vi "filterField.vi"(4 "Lado":enum16{"Esquerdo", "Direito"}(ring)=enum."Direito" caption="Enum", 5 "ignora esquerda?":bool=TRUE, 6 "Time":enum16{"Azul", "Amarelo"}(ring) caption="Enum", 7 "ignora lado?":bool=TRUE, 8 "error in (no error)":errorcluster, 9 "Estimador":T6, 10 "SSL UDP RX":T7, 11 "Vision in":refnum<class "Vision.lvclass">) -> (0 "error out":errorcluster, 1 "RX":bool, 2 "Frame and Field Size out":T1 {"Detection Frame Out"."robots_blue"."height" format="%+4.3f"; "Detection Frame Out"."robots_blue"."pixel_y" format="%+4.3f"; "Detection Frame Out"."robots_blue"."pixel_x" format="%+4.3f"; "Detection Frame Out"."robots_blue"."orientation" format="%+4.3f"; "Detection Frame Out"."robots_blue"."y" format="%+4.3f"; "Detection Frame Out"."robots_blue"."confidence" format="%4.3f"; "Detection Frame Out"."robots_blue"."x" format="%+4.3f"; "Detection Frame Out"."robots_yellow"."height" format="%+4.3f"; "Detection Frame Out"."robots_yellow"."pixel_y" format="%+4.3f"; "Detection Frame Out"."robots_yellow"."pixel_x" format="%+4.3f"; "Detection Frame Out"."robots_yellow"."orientation" format="%+4.3f"; "Detection Frame Out"."robots_yellow"."y" format="%+4.3f"; "Detection Frame Out"."robots_yellow"."confidence" format="%4.3f"; "Detection Frame Out"."robots_yellow"."x" format="%+4.3f"}, 3 "Vision out":refnum<class "Vision.lvclass">)   [LabVIEW 2018, in "Vision.lvclass"]
uses:
  Vision.lvclass
  vision_control.ctl
  Old vision/Controls/Estimadores.ctl
  Old vision/Controls/SSL Field State.ctl
  Old vision/Controls/SSL Detection Frame.ctl
  Old vision/Controls/SSL Detection Robot.ctl
  <vilib>/Analysis/Matrix/Datatypes/RealMatrix.ctl
  Old vision/Controls/SSL Detection Ball.ctl
  <vilib>/Analysis/Matrix/NI_Matrix.lvlib
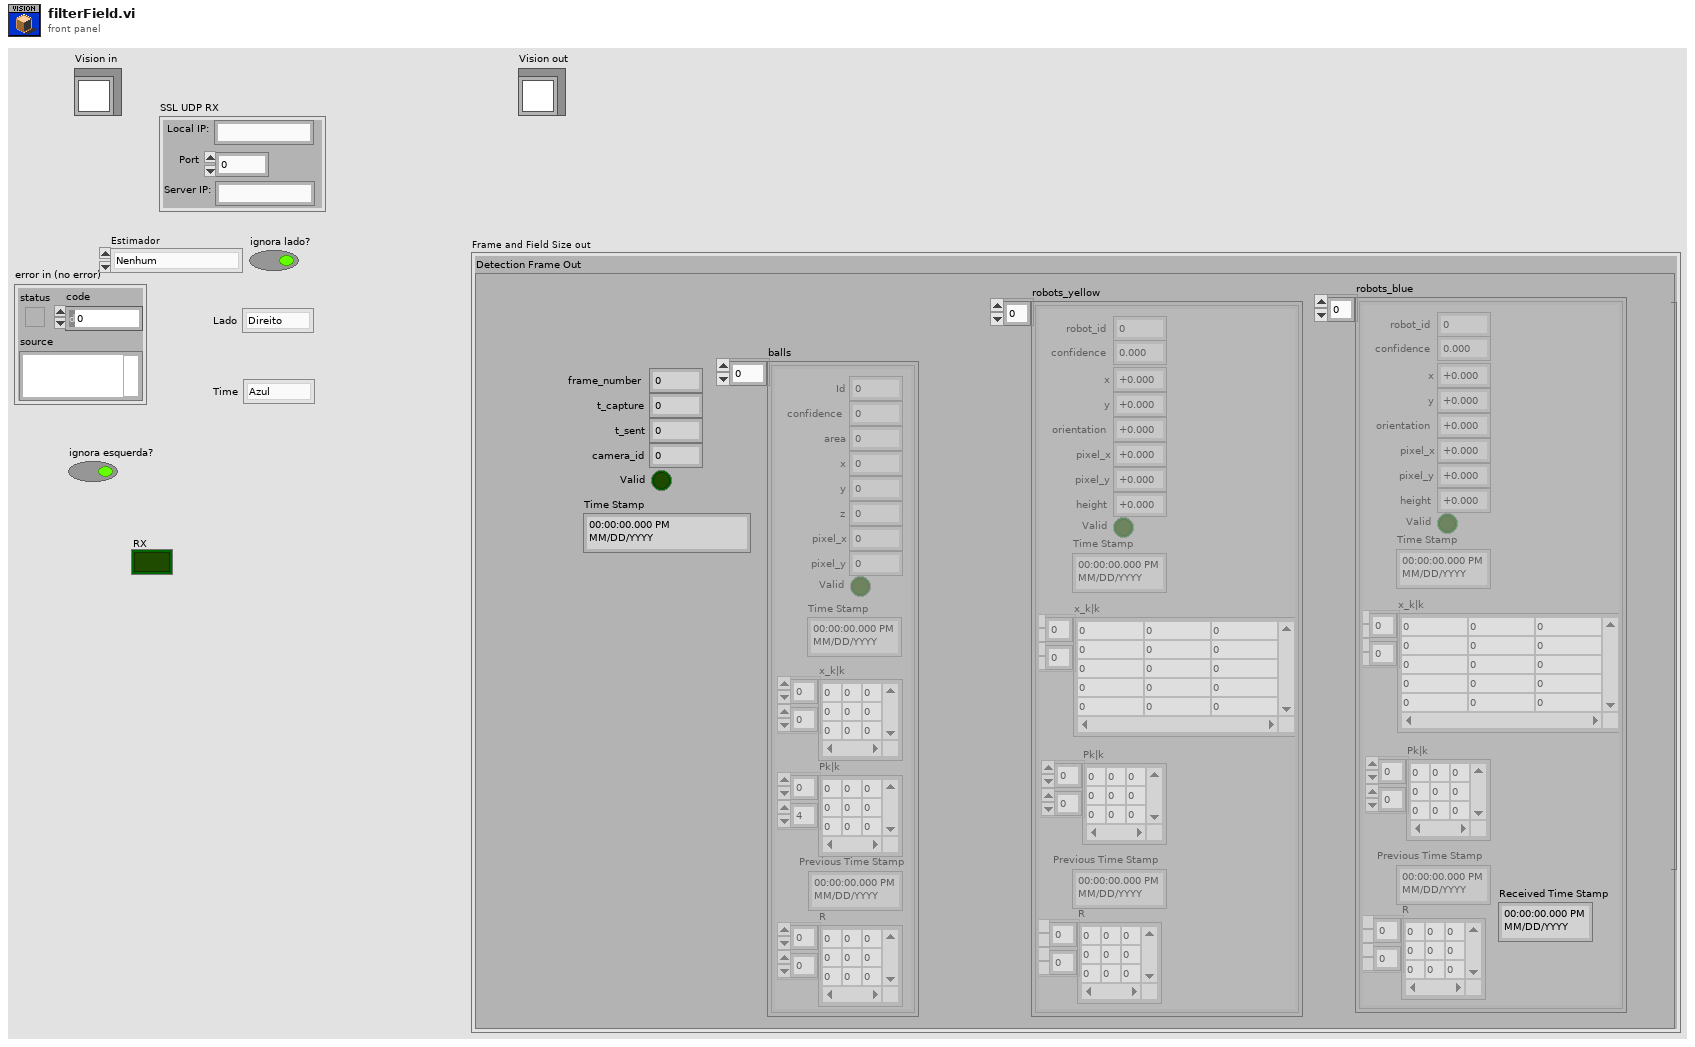
[diagram p1: front panel]
types:
  T1 = typedef "SSL Field State.ctl" = cluster{"Detection Frame Out":T2, "Field Size Out":cluster{"line_width":u32, "field_length":u32, "field_width":u32, "boundary_width":u32, "referee_width":u32, "goal_width":u32, "goal_depth":u32, "goal_wall_width":u32, "center_circle_radius":u32, "defense_radius":u32, "defense_stretch":u32, "free_kick_from_defense_dist":u32, "penalty_spot_from_field_line_dist":u32, "penalty_line_from_spot_dist":u32}, "Received Time Stamp":timestamp}
  T2 = typedef "SSL Detection Frame.ctl" = cluster{"frame_number":u32, "t_capture":dbl, "t_sent":dbl, "camera_id":u32, "robots_yellow":T3[], "robots_blue":T3[], "balls":T5[], "Valid":bool, "Time Stamp":timestamp}
  T3 = typedef "SSL Detection Robot.ctl" = cluster{"x":sgl, "robot_id":u32, "confidence":sgl, "y":sgl, "orientation":sgl, "pixel_x":sgl, "pixel_y":sgl, "height":sgl, "Valid":bool, "Time Stamp":timestamp, "x_k|k":T4, "Pk|k":T4, "Previous Time Stamp":timestamp, "R":T4}
  T4 = typedef "NI_Matrix.lvlib/RealMatrix.ctl" = dbl[][]
  T5 = typedef "SSL Detection Ball.ctl" = cluster{"x":sgl, "area":u32, "confidence":sgl, "y":sgl, "z":sgl, "pixel_x":sgl, "pixel_y":sgl, "Valid":bool, "Time Stamp":timestamp, "x_k|k":T4, "Pk|k":T4, "Id":u32, "Previous Time Stamp":timestamp, "R":T4}
  T6 = typedef "Estimadores.ctl" = enum16{"Nenhum", "Simples", "Kalman"}
  T7 = typedef "vision_control.ctl" = cluster{"Local IP:":string, "Port":i32, "Server IP:":string}
  T8 = cluster{"line_width":u32, "field_length":u32, "field_width":u32, "boundary_width":u32, "referee_width":u32, "goal_width":u32, "goal_depth":u32, "goal_wall_width":u32, "center_circle_radius":u32, "defense_radius":u32, "defense_stretch":u32, "free_kick_from_defense_dist":u32, "penalty_spot_from_field_line_dist":u32, "penalty_line_from_spot_dist":u32}
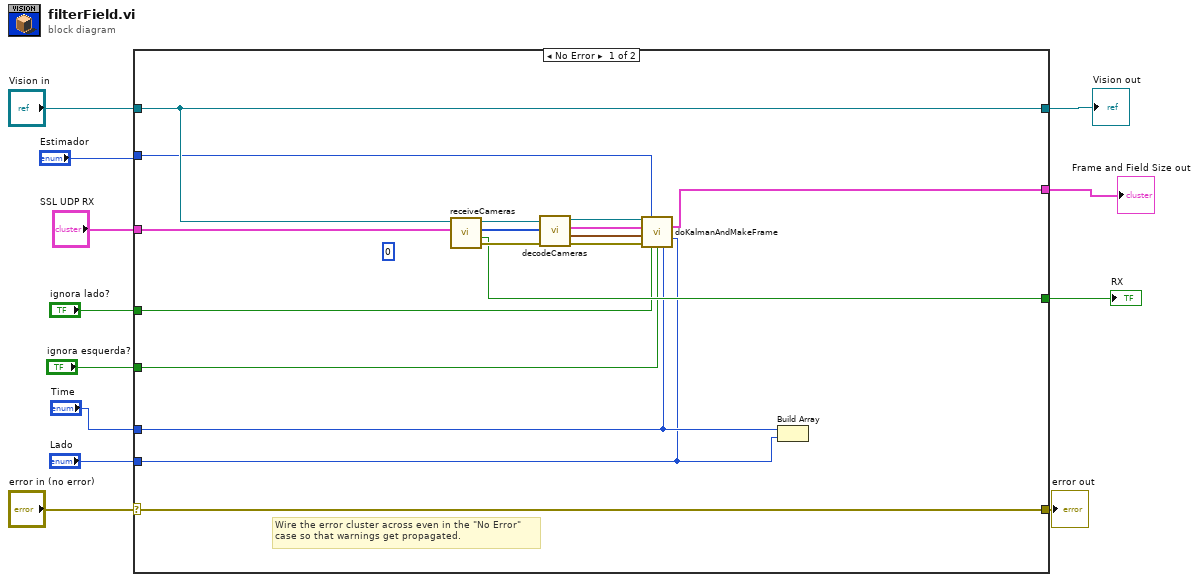
[diagram p0: block diagram]
diagram:
  n1 = case shown="No Error" "error in (no error)" {
    selector: "error in (no error)" -> [w29 w31]
    tunnel: [w29 w31] -> w11
    tunnel: [w18 w30] -> w9
    tunnel: "Vision in" -> [w18 w30]
    tunnel: [w21 _] -> w8
    tunnel: [w20 _] -> w7
    tunnel: "SSL UDP RX" -> [w19 _]
    tunnel: "ignora lado?" -> [w17 _]
    tunnel: "ignora esquerda?" -> [w16 _]
    tunnel: "Time" -> [w15 _]
    tunnel: "Lado" -> [w14 _]
    tunnel: "Estimador" -> [w13 _]
    frame No Error {
      (unwired) u32 0 ("milliseconds to wait")
      # "Wire the error cluster across even in the \"No Error\"\ncase so that warnings get propagated."
      n2 = call "receiveCameras.vi"("Cluster"=w19, "Vision in"=w18) -> ("error out"=w26:errorcluster, "RX"=w20:bool, "data camera out"=w27:u8[], "Vision out"=w28:refnum<class "Vision.lvclass">)  [unwired: 5 in]
      n3 = call "decodeCameras.vi"("error in (no error)"=w26, "unsigned byte array"=w27, "Vision in"=w28) -> ("error out"=w22:errorcluster, "Field Size"=w23:T8, "Detection Frame"=w24:T2, "Vision out"=w25:refnum<class "Vision.lvclass">)  [unwired: 5 in]
      n4 = call "doKalmanAndMakeFrame.vi"("Vision in"=w25, "Estimador"=w13, "Detection Frame"=w24, "Field Size"=w23, "Lado"=w14, "error in (no error)"=w22, "ignora lado?"=w17, "ignora esquerda?"=w16, "Time"=w15) -> ("Frame and Field Size out"=w21:T1)  [unwired: 4 in, 2 out]
      n5 = Build Array(w15, w14) -> ()  [unwired: 1 out]
    }
    frame Error {
    }
  }
  "error out" <- w11
  "Vision out" <- w9
  "Frame and Field Size out" <- w8
  "RX" <- w7
